vi "Python TCP Connection Handler.vi"(9 "Additional Data":variant, 10 "connection ID":T2, 11 "TCP Server Reference":T1) -> ()   [LabVIEW 2013, in "JKI_Python_Bridge_for_LV.lvlib" / "Server.lvclass"]
uses:
  Server.lvclass
  <vilib>/addons/_JKI.lib/_jki_lib_tcp_server.llb/TCP Server Connection Session ID Cluster__jki_lib_tcp_server.ctl
  <vilib>/addons/_JKI.lib/_jki_lib_tcp_server.llb/TCP Server Object RefNum__jki_lib_tcp_server.ctl
  <vilib>/addons/_JKI.lib/_jki_lib_tcp_server.llb/TCP Server Object RefNum - Enum__jki_lib_tcp_server.ctl
  PythonResponseType.ctl
  Type Definitions/Python Class Data - Cluster.ctl
  PyObject/PyObject.lvclass/PyObject.ctl
  <vilib>/addons/_JKI.lib/_JKI_lib_Python_Data_Tools.llb/LabVIEW Data to Python String (String)__jki_lib_python_data_tools.vi
  <vilib>/addons/_JKI.lib/_JKI_lib_Python_Data_Tools.llb/LabVIEW Data to Python String (Variant)__jki_lib_python_data_tools.vi
  <vilib>/Utility/error.llb/DialogType.ctl
  PyObject/PyObject.lvclass
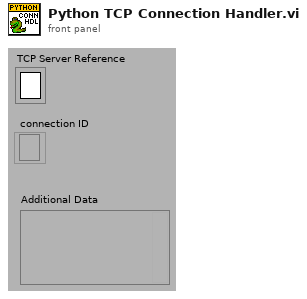
[diagram p1: front panel]
types:
  T1 = typedef "TCP Server Object RefNum__jki_lib_tcp_server.ctl" = refnum<k1>
  T2 = typedef "TCP Server Connection Session ID Cluster__jki_lib_tcp_server.ctl" = refnum<k5>
  T3 = enum16{"Standard", "Buffered", "CRLF", "Immediate"}
  T4 = typedef "JKI_Python_Bridge_for_LV.lvlib/Server.lvclass/PythonResponseType.ctl" = enum16{"ERRor", "OK", "NEXT"}
  T5 = typedef "JKI_Python_Bridge_for_LV.lvlib/Server.lvclass/Python Class Data - Cluster.ctl" = cluster{"Name":string, "Functions":cluster{"Name":string, "Arguments":string[], "Documentation":string}[]}
  T6 = typedef "JKI_Python_Bridge_for_LV.lvlib/Server.lvclass/Python Node.ctl" = cluster{"Name":string, "Python Method Call":refnum<user-event>, "Call Handle":refnum<class "PyObject.lvclass">}
  T7 = cluster{"Name":string, "Arguments":string[], "Documentation":string}[]
  T8 = typedef "JKI_Python_Bridge_for_LV.lvlib/Server.lvclass/Python Response - Cluster.ctl" = cluster{"Python Response":variant, "error out":errorcluster}
  T9 = typedef "DialogType.ctl" = u16
  T10 = cluster{"code out":i32, "delimited string":string, "delimited string":string}
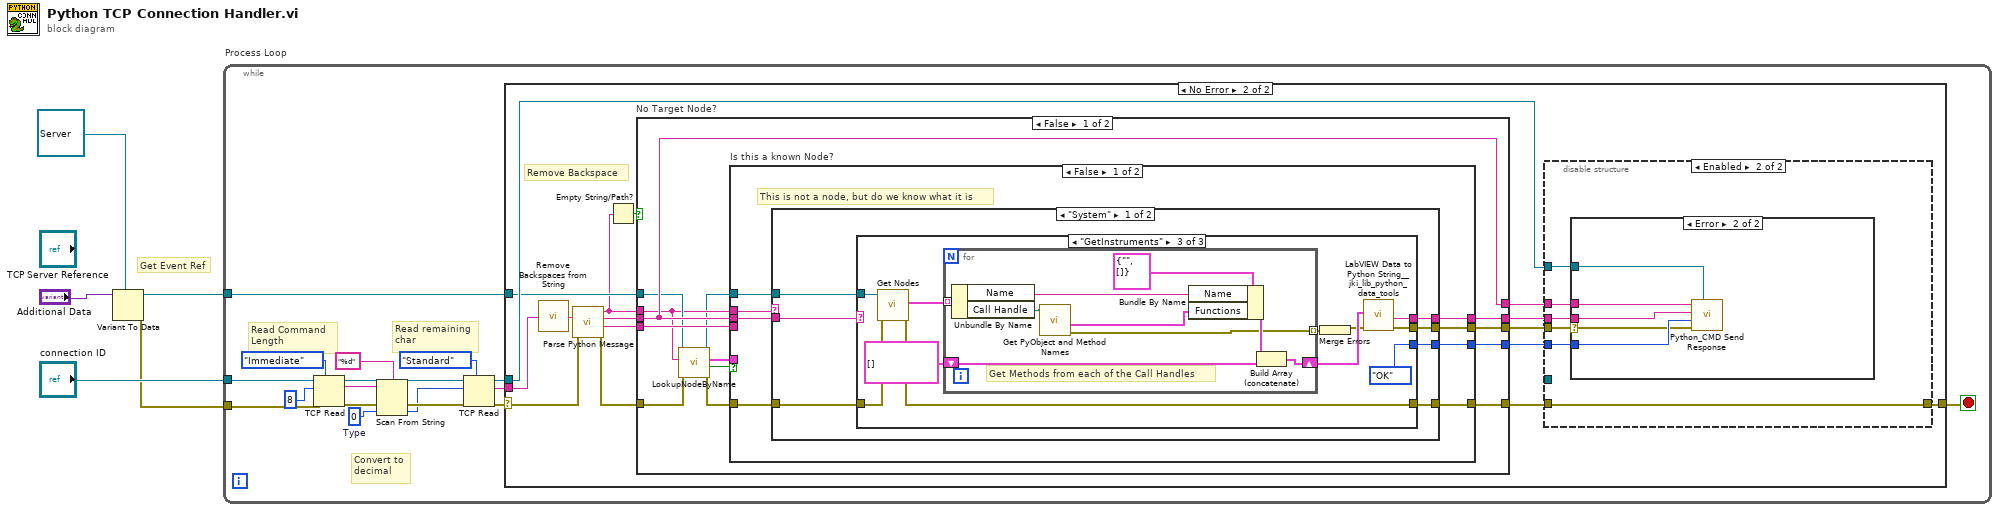
[diagram p0: block diagram]
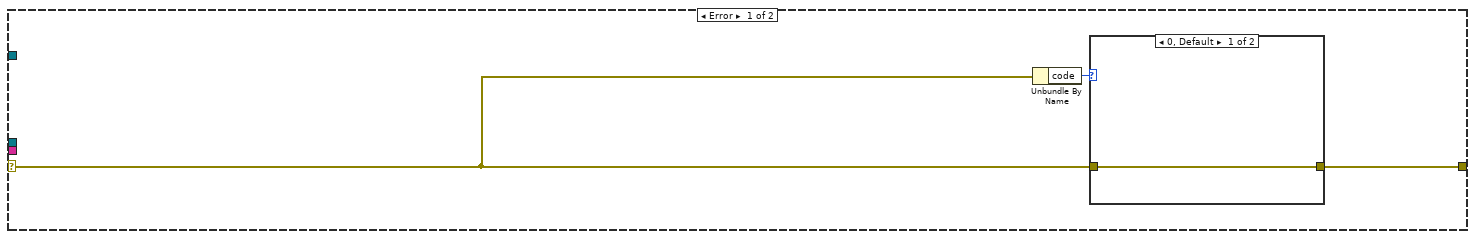
[diagram p2: hidden frame]
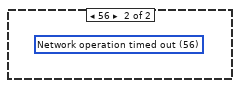
[diagram p3: hidden frame]
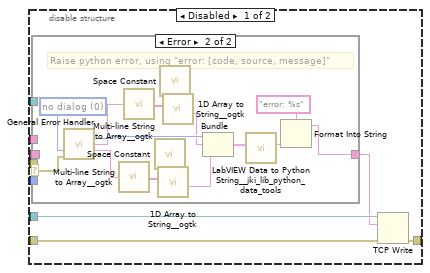
[diagram p4: hidden frame]
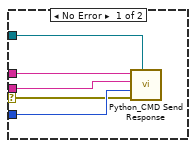
[diagram p6: hidden frame]
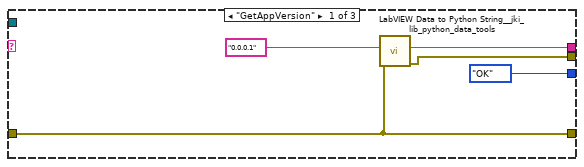
[diagram p7: hidden frame]
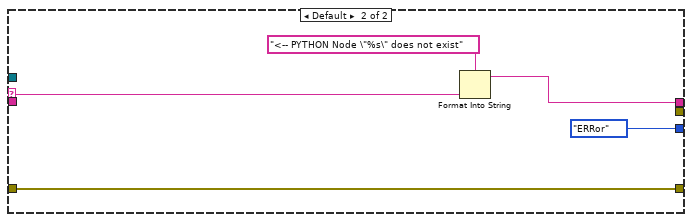
[diagram p9: hidden frame]
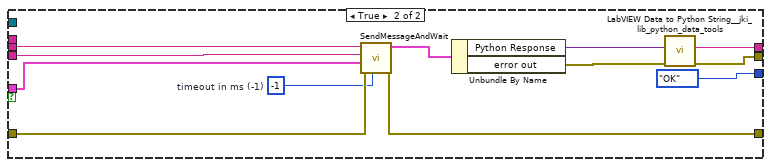
[diagram p10: hidden frame]
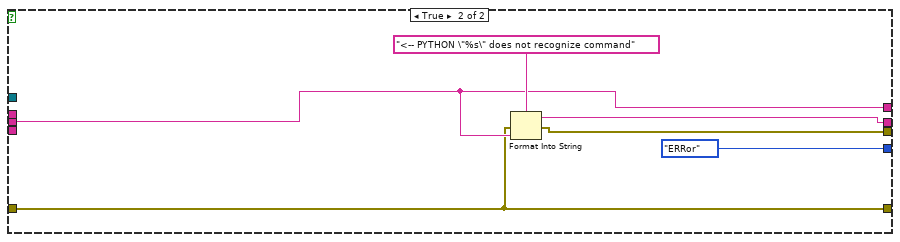
[diagram p11: hidden frame]
diagram:
  # "Get Event Ref"
  n1 = Variant To Data(type=refnum<class "Server.lvclass"> refnum ("JKI_Python_Server in"), Variant="Additional Data") -> (data=w2:refnum<class "Server.lvclass">, error out=w1:errorcluster)  [unwired: 1 in]
  n2 = while "Process Loop" {
    tunnel: "connection ID" -> [w17]
    tunnel: w2 -> [w7]
    tunnel: w1 -> [w6]
    stop <- w22 stop-if-true
    w9 = 0  # Type
    # "Read remaining\nchar"
    # "Convert to\ndecimal"
    # "Read Command\nLength"
    n3 = TCP Read(connection ID=w17, bytes to read=8, error in (no error)=w6, 7:T3."Immediate" ("mode (standard)")) -> (connection ID out=w16:T2, data out=w13:string, error out=w14:errorcluster)  [unwired: 1 out]
    n4 = Scan From String(format string="%d", input string=w13, error in=w14, default 1=w9) -> (error out=w12:errorcluster, output 1=w8:i32)  [unwired: 1 in, 2 out]
    n5 = TCP Read(connection ID=w16, bytes to read=w8, error in (no error)=w12, 7:T3."Standard" ("mode (standard)")) -> (connection ID out=w18:T2, data out=w19:string, error out=w20:errorcluster)  [unwired: 1 out]
    n6 = case shown="No Error" w20 {
      selector: w20 -> [w24 w30]
      tunnel: w18 -> [_ w33]
      tunnel: w19 -> [_ w28]
      tunnel: [w23 w42] -> w22
      tunnel: w7 -> [_ w32]
      frame Error {
        n7 = Unbundle By Name(w24) -> ("code"=w25:i32)
        n8 = case shown="0, Default" w25 {
          tunnel: w24 -> [w26 _]
          tunnel: [w26 _] -> w23
          frame 0, Default {
          }
          frame 56 {
            (unwired) 56 items=["No error", "Argument error", "Memory is full", "Out of zone", "End of file", "File already open", "Generic file I/O error", "File not found", "File permission error", "Disk is full", "Duplicate path", "Too many files open", "System feature not enabled", "Resource file not found", "Cannot add resource", "Resource not found", "Image not found", "Image memory error", "Pen does not exist", "Config type invalid", "Config token not found", "Config parse error", "Config memory error", "Bad external code format", "Bad external code offset", "External code not present", "Null window", "Destroy window error", "Null menu", "Print aborted", "Bad print record", "Print driver error", "Windows error during printing", "Memory error during printing", "Print dialog error", "Generic print error", "Invalid device refnum", "Device not found", "Device parameter error", "Device unit error", "Cannot open device", "Device call aborted", "Generic error", "Cancelled by user", "Object ID too low", "Object ID too high", "Object not in heap", "Unknown heap", "Unknown object (invalid DefProc)", "Unknown object (DefProc not in table)", "Message out of range", "Invalid (null) method", "Unknown message", "Manager call not supported", "Bad address", "Network operation in progress", "Network operation timed out", "Connection is busy", "Network attribute not supported", "Network error", "Address in use", "System out of memory", "Connection aborted", "Connection refused", "Not connected", "Already connected", "Connection closed", "Initialization error (interapplication manager)", "Bad occurrence", "Wait on unbound occurrence handler", "Occurrence queue overflow", "Datalog type conflict", "Unused", "Unrecognized type (interapplication manager)", "Memory corrupt", "Failed to make temporary DLL", "Old CIN version", "Drag socket not found", "Failed to load drop-object", "Failed to register OLE object", "Failed to release OLE object", "Format specifier type mismatch", "Unknown format specifier", "Too few format specifiers", "Too many format specifiers", "Scan failed", "Newer CIN version", "Error converting to variant", "Runtime menu error", "Password tampered", "Variant attribute not found", "Incompatible variant data type", "Event data is not available", "Event Store is not present", "Occurrence is not found", "Event Queue is not created", "Event info is not available", "Refnum passed is NULL", "Error retrieving Class GUID", "Error retrieving CoClass GUID", "Error retrieving TypeLib GUID.", "Bad built application magic bytes.", "Specific driver is different from the specific driver associated with the Logical Name.", "There is no session opened to the class driver.", "Max Error", "MAX - Error with config objects", "MAX - Error loading configuration", "MAX - Group not supported"]
          }
        }
      }
      frame No Error {
        # "Remove Backspace"
        n9 = call "Remove Backspaces from String.vi"("String in"=w28) -> ("String out"=w27:string)  [unwired: 4 in]
        n10 = call "Parse Python Message.vi"("error in"=w30, "Python Message"=w27) -> ("error out"=w29:errorcluster, "Argument String"=w38:string, "PYTHON Command"=w39:string, "PYTHON Node Name"=w31:string)  [unwired: 6 out]
        n11 = Empty String/Path?(string/path=w31) -> (empty?=w37:bool)
        n12 = case "No Target Node?" shown="False" w37 {
          tunnel: [w92 w151] -> w41
          tunnel: [w91 w155] -> w40
          tunnel: w29 -> [w85 w151]
          tunnel: w39 -> [w89 w152]
          tunnel: w38 -> [w90 _]
          tunnel: [w87 w156] -> w36
          tunnel: [w89 w152] -> w35
          tunnel: [w88 PythonResponseType."ERRor" ("Response Type")] -> w34
          tunnel: w32 -> [w83 _]
          tunnel: w31 -> [w81 _]
          frame False {
            n13 = call "LookupNodeByName.vi"("error in (no error)"=w85, "Python Node Name"=w81, "Server in"=w83) -> ("error out"=w84:errorcluster, "Found?"=w86:bool, "PYTHON Node"=w82:T6, "Server out"=w80:refnum<class "Server.lvclass">)  [unwired: 5 in]
            n14 = case "Is this a known Node?" shown="False" w86 {
              tunnel: [w95 w150] -> w92
              tunnel: [w98 w147] -> w91
              tunnel: w84 -> [w96 w146]
              tunnel: w90 -> [_ w145]
              tunnel: w89 -> [w99 w144]
              tunnel: [w97 PythonResponseType."OK" ("Response Type")] -> w88
              tunnel: [w93 w142] -> w87
              tunnel: w82 -> [_ w141]
              tunnel: w81 -> [w100 _]
              tunnel: w80 -> [w94 _]
              frame False {
                # "This is not a node, but do we know what it is"
                n15 = case shown="\"System\"" w100 {
                  selector: w100 -> [_ w136]
                  tunnel: w99 -> [w105 _]
                  tunnel: [w107 w138] -> w98
                  tunnel: [w104 PythonResponseType."ERRor" ("Response Type")] -> w97
                  tunnel: w96 -> [w103 w134]
                  tunnel: [w106 w134] -> w95
                  tunnel: w94 -> [w102 _]
                  tunnel: [w101 _] -> w93
                  frame "System" {
                    n16 = case shown="\"GetInstruments\"" w105 {
                      tunnel: [w110 _ w117] -> w107
                      tunnel: w103 -> [w108 w113 w122]
                      tunnel: [w108 w113 w116] -> w106
                      tunnel: [PythonResponseType."OK" ("Response Type") _ PythonResponseType."OK" ("Response Type")] -> w104
                      tunnel: w102 -> [_ _ w123]
                      tunnel: [w109 _ w119] -> w101
                      frame "GetAppVersion" {
                        n17 = call-poly <vilib>:"LabVIEW Data to Python String__jki_lib_python_data_tools.vi"("error in (no error)"=w108, "LabVIEW Data"="0.0.0.1" ("Python String")) -> ("error out"=w109:errorcluster, "Python String"=w110:string)  [unwired: 8 in]
                      }
                      frame Default {
                      }
                      frame "GetInstruments" {
                        n18 = call "Get Nodes.vi"("error in (no error)"=w122, "JKI_Python_Server in"=w123) -> ("error out"=w116:errorcluster, "Nodes"=w121:T6[])  [unwired: 7 in, 1 out]
                        n19 = for {
                          tunnel: w121 -> [w133] mode=indexing
                          shift-right: [w132] -> w118
                          shift-left: T5[] [] -> [w131]
                          tunnel: [w126] -> w115 mode=indexing
                          # "Get Methods from each of the Call Handles"
                          n20 = Unbundle By Name(w133) -> ("Name"=w129:string, "Call Handle"=w130:refnum<class "PyObject.lvclass">)
                          n21 = call "Get PyObject and Method Names.vi"("Node in"=w130) -> ("error out"=w126:errorcluster, "Functions"=w125:T7)  [unwired: 7 in, 2 out]
                          n22 = Bundle By Name(cluster=T5 {"Name"="", "Functions"=[]} ("Python Class Data"), "Name"=w129, "Functions"=w125) -> (w127:T5)
                          n23 = Build Array (concatenate)(w127, w131) -> (w132:T5[])
                        }
                        n24 = Merge Errors(w115) -> (w114:errorcluster)
                        n25 = call-poly <vilib>:"LabVIEW Data to Python String__jki_lib_python_data_tools.vi"("error in (no error)"=w114, "LabVIEW Data"=w118) -> ("error out"=w119:errorcluster, "Python String"=w117:string)  [unwired: 8 in]
                      }
                    }
                  }
                  frame Default {
                    n26 = Format Into String(format string="<-- PYTHON Node \"%s\" does not exist", w136) -> (resulting string=w138:string)  [unwired: 2 in, 1 out]
                  }
                }
              }
              frame True {
                w139 = -1  # timeout in ms (-1)
                n27 = call "SendMessageAndWait.vi"("timeout in ms (-1)"=w139, "error in (no error)"=w146, "PYTHON Node"=w141, "Argument String"=w145, "PYTHON Command"=w144) -> ("error out"=w150:errorcluster, "Reply"=w140:T8)  [unwired: 5 in]
                n28 = Unbundle By Name(w140) -> ("Python Response"=w148:variant, "error out"=w149:errorcluster)
                n29 = call-poly <vilib>:"LabVIEW Data to Python String__jki_lib_python_data_tools.vi"("error in (no error)"=w149, "LabVIEW Data"=w148) -> ("error out"=w142:errorcluster, "Python String"=w147:string)  [unwired: 8 in]
              }
            }
          }
          frame True {
            n30 = Format Into String(format string="<-- PYTHON \"%s\" does not recognize command", error in=w151, w152) -> (resulting string=w155:string, error out=w156:errorcluster)  [unwired: 1 in]
          }
        }
        n31 = disable-structure shown="Enabled" {
          disable-tunnel: _ -> [w47 _]
          disable-tunnel: [w46 w69] -> w42
          disable-tunnel: w41 -> [w44 w69]
          disable-tunnel: w40 -> [w43 w68]
          disable-tunnel: w36 -> [_ w64]
          disable-tunnel: w33 -> [_ w67]
          disable-tunnel: w35 -> [_ w66]
          disable-tunnel: w34 -> [_ w65]
          frame Disabled {
            n32 = case shown="Error" {
              selector: _ -> [_ w63]
              tunnel: w43 -> [w48 _]
              tunnel: [w48 w57] -> w45
              frame No Error {
              }
              frame Error {
                w62 = T9 0 items=["no dialog", "OK message", "continue or stop message", "OK message + warnings", "continue/stop + warnings"] ("type of dialog (OK msg:1)")
                # "Raise python error, using \"error: [code, source, message]\""
                n33 = call <vilib>:"General Error Handler.vi"("type of dialog (OK msg:1)"=w62, "error in (no error)"=w63) -> ("code out"=w61:i32, "source out"=w50:string, "message"=w56:string)  [unwired: 11 out]
                n34 = call <userlib>:"Multi-line String to Array__ogtk.vi"("string"=w56) -> ("lines"=w55:string[])
                n35 = call <userlib>:"Multi-line String to Array__ogtk.vi"("string"=w50) -> ("lines"=w51:string[])
                n36 = call <vilib>:"Space Constant.vi"() -> ("String"=w54:string)
                n37 = call <userlib>:"1D Array to String__ogtk.vi"("delimiter (Tab)"=w54, "Array of Strings"=w55) -> ("delimited string"=w53:string)  [unwired: 9 out]
                n38 = call <vilib>:"Space Constant.vi"() -> ("String"=w52:string)
                n39 = call <userlib>:"1D Array to String__ogtk.vi"("delimiter (Tab)"=w52, "Array of Strings"=w51) -> ("delimited string"=w49:string)  [unwired: 9 out]
                n40 = Bundle("code out"=w61, "delimited string"=w49, "delimited string"=w53) -> (w60:T10)  [unwired: 1 out]
                n41 = call-poly <vilib>:"LabVIEW Data to Python String__jki_lib_python_data_tools.vi"("LabVIEW Data"=w60) -> ("Python String"=w59:string)  [unwired: 9 in, 1 out]
                n42 = Format Into String(format string="error: %s", w59) -> (resulting string=w57:string)  [unwired: 2 in, 1 out]
              }
            }
            n43 = TCP Write(connection ID=w47, data in=w45, error in (no error)=w44) -> (error out=w46:errorcluster)  [unwired: 3 out]
          }
          frame Enabled {
            n44 = case shown="Error" w64 {
              selector: w64 -> [w70 w75]
              tunnel: w68 -> [w74 w79]
              tunnel: w67 -> [w73 w78]
              tunnel: w66 -> [w72 w77]
              tunnel: w65 -> [w71 w76]
              frame No Error {
                n45 = call "Python_CMD Send Response.vi"("TCP Connection ID"=w73, "non-fatal error"=w70, "Response Type"=w71, "Response"=w74, "PYTHON Command String"=w72) -> ()  [unwired: 6 in, 1 out]
              }
              frame Error {
                n46 = call "Python_CMD Send Response.vi"("TCP Connection ID"=w78, "non-fatal error"=w75, "Response Type"=w76, "Response"=w79, "PYTHON Command String"=w77) -> ()  [unwired: 6 in, 1 out]
              }
            }
          }
        }
      }
    }
  }
